vi "GetFPSrange.vi"(8 "error in":errorcluster, 11 "camera.nit_c in":refnum<class "camera.lvclass">) -> (0 "error out":errorcluster, 1 "max":dbl, 2 "min":dbl, 3 "current":dbl)   [LabVIEW 2020, in "camera.lvclass"]
uses:
  camera.lvclass
  camera.lvclass/camera.ctl
  lib/O-PL.dll
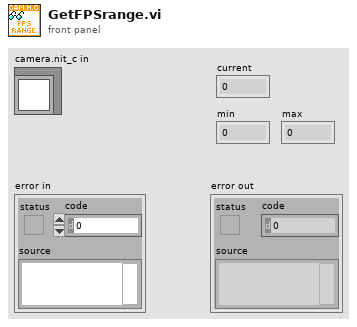
[diagram p1: front panel]
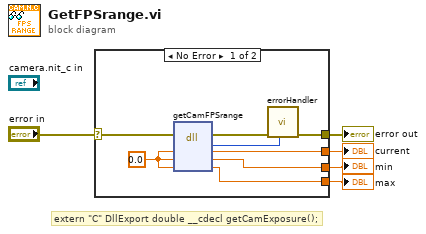
[diagram p0: block diagram]
diagram:
  # "extern \"C\" DllExport double __cdecl getCamExposure();"
  n1 = case shown="No Error" "error in" {
    selector: "error in" -> [w13 _]
    tunnel: [w7 _] -> w5
    tunnel: [w12 _] -> w4
    tunnel: [w11 _] -> w2
    tunnel: [w9 _] -> w1
    frame No Error {
      w10 = 0.0 ("current")
      n2 = dll-call lib="D:/UNSW - New/v0.8.3/lib/O-PL.dll" fn="getCamFPSrange"(error in=w13, "current"=w10, "Min"=w10, "Max"=w10) -> (error out=w8:errorcluster, "return type"=w6:i32, "current"=w9:dbl, "Min"=w12:dbl, "Max"=w11:dbl)  [unwired: 2 in, 1 out]
      n3 = call "errorHandler.vi"("code"=w6, "error in"=w8) -> ("error out"=w7:errorcluster)  [unwired: 9 in]
    }
    frame Error {
    }
  }
  "error out" <- w5
  "min" <- w4
  "max" <- w2
  "current" <- w1
